vi "SetConversionFactorsAndSetupLogger.vi"(8 "error out 2":errorcluster, 11 "Protocol_Generic out 2":refnum<class "Protocol_Logging.lvclass">) -> (0 "error out":errorcluster, 3 "Protocol_Generic out":refnum<class "Protocol_Logging.lvclass">)   [LabVIEW 2011, in "Protocol_Logging.lvclass"]
uses:
  Protocol_Logging.lvclass
  Protocol_Logging.lvclass/Protocol_Logging.ctl
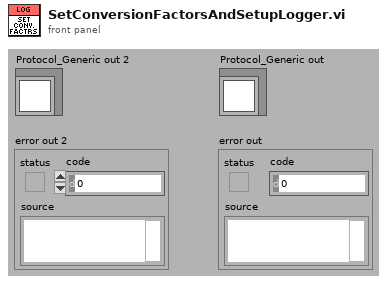
[diagram p1: front panel]
types:
  T1 = cluster{"Axis Information":cluster{"Device ID":i32, "Device Name":string, "Device Type":i32}[], "Axis Selector":i32[], "Control Modes out":u16[], "error out":errorcluster, "Channel Data":cluster{"Name":string, "Type":i32, "SI Full Scale":dbl, "Full Scale":dbl, "Units String":string, "Display Format":string, "Gauge Length":dbl}[][]}
  T2 = cluster{"Device ID":i32, "Device Name":string, "Device Type":i32}[]
  T3 = cluster{"Name":string, "Type":i32, "SI Full Scale":dbl, "Full Scale":dbl, "Units String":string, "Display Format":string, "Gauge Length":dbl}[][]
  T4 = cluster{"Sample interval - ms (2)":dbl, "Buffer Length (1000)":i32, "No. of Buffers (0)":i32}
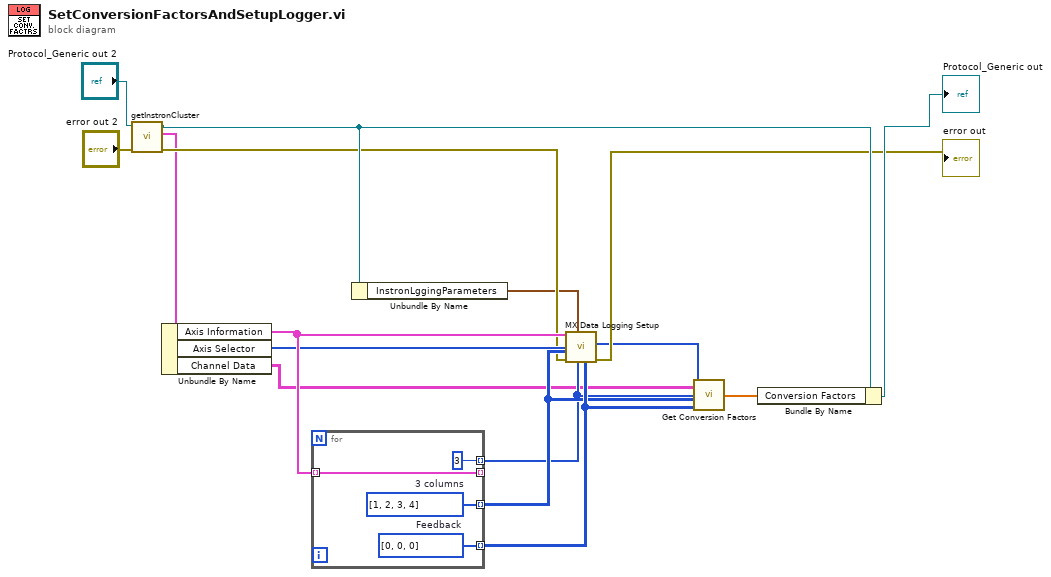
[diagram p0: block diagram]
diagram:
  n1 = call-dynamic "getInstronCluster.vi"("error in (no error)"="error out 2", "Protocol_Generic in"="Protocol_Generic out 2") -> ("error out"=w7:errorcluster, "InstronCluster"=w6:T1, "Protocol_Generic out"=w10:refnum<class "Protocol_Logging.lvclass">)  [unwired: 7 in]
  n2 = Unbundle By Name(w6) -> ("Axis Information"=w13:T2, "Axis Selector"=w9:i32[], "Channel Data"=w2:T3)
  n3 = for {
    tunnel: [w20] -> w15 mode=indexing
    tunnel: [w19] -> w16 mode=indexing
    tunnel: [3] -> w14 mode=indexing
    tunnel: [w17] -> _ mode=indexing
    tunnel: w13 -> [w17] mode=indexing
    w19 = i32[] [0, 0, 0]  # Feedback
    w20 = i32[] [1, 2, 3, 4]  # 3 columns
  }
  n4 = Unbundle By Name(w10) -> ("InstronLggingParameters"=w3:T4)
  n5 = call "MX Data Logging Setup.vi"("Column Types"=w16, "Number of Columns"=w14, "Interval/Buffer Parameters"=w3, "error in (no error)"=w7, "Column Channels"=w15, "Axis Selector"=w9, "Axis Information"=w13) -> ("error out"=→"error out":errorcluster, "Axis Selector copy"=w1:i32[])  [unwired: 2 out]
  n6 = call "Get Conversion Factors.vi"("Axis Selector"=w1, "Channel Data"=w2, "Column Channels"=w15, "Column Types"=w16, "Number of Columns"=w14) -> ("Conversion Factors"=w12:dbl[])
  n7 = Bundle By Name(cluster=w10, "Conversion Factors"=w12) -> (→"Protocol_Generic out":refnum<class "Protocol_Logging.lvclass">)
